vi "글로벌플라이트플랜.vi"() -> ()   [LabVIEW 2014]
panel:
  out "기록":string[](array[string])
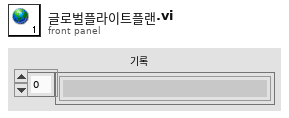
[diagram p1: front panel]
diagram:
